vi "opt_power.vi"(11 "file path 2":path=path "C:/luminartech/ManufacturingTools/TS_Automation/Programs/Labview/bring_up/find_opt_power/opt_power_resp.txt") -> (3 "opt_power":dbl)   [LabVIEW 2018]
panel:
  out "size(s)":i32
  out "text 2":string[](array[string])
  out "line 2":string
  out "data table":dbl[][](array[numeric])
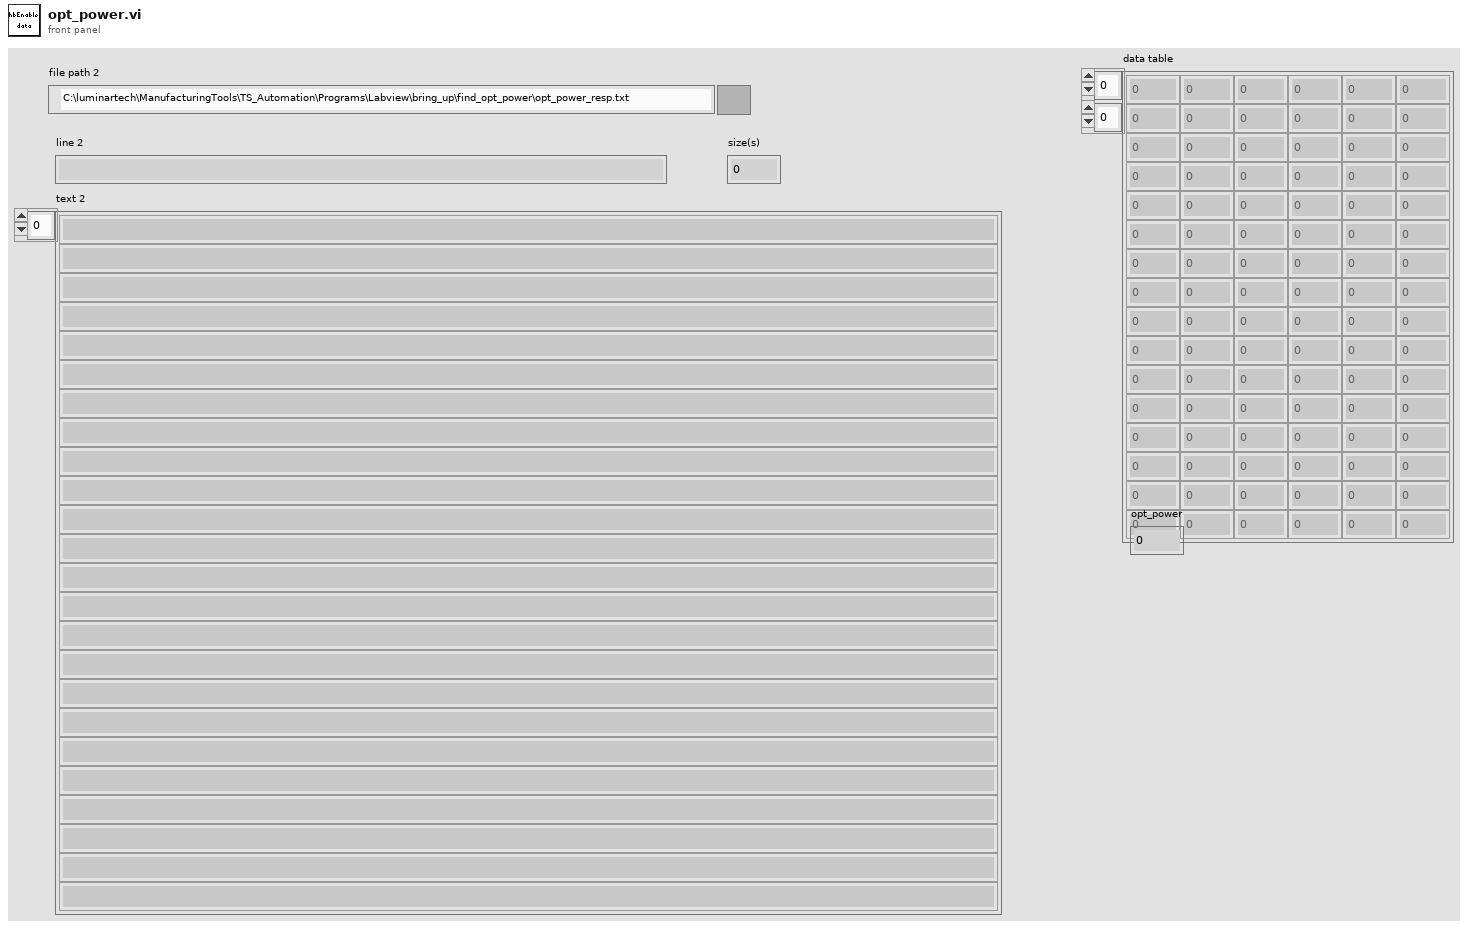
[diagram p1: front panel]
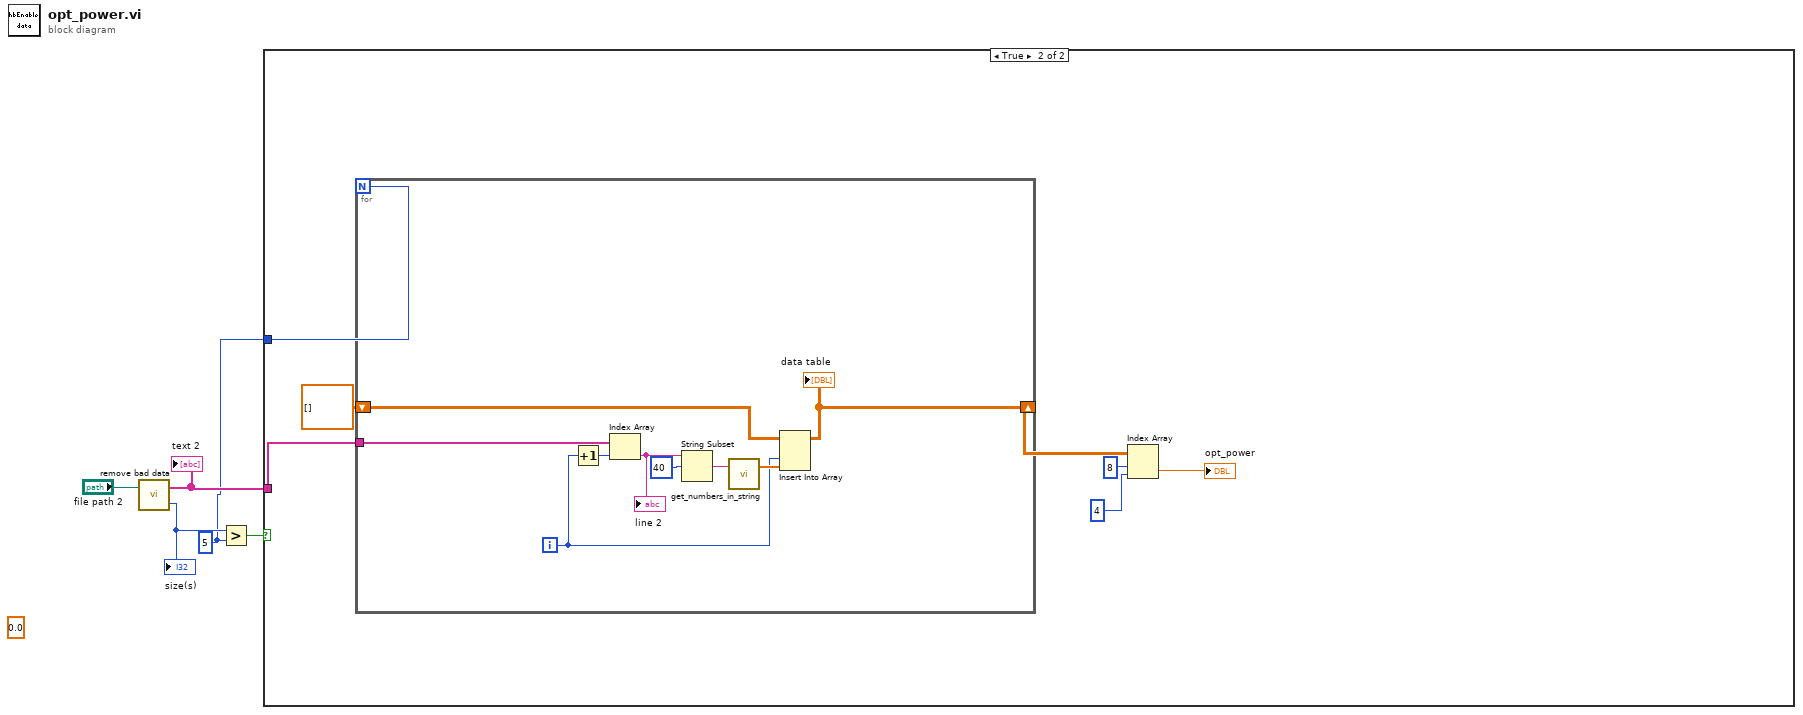
[diagram p0: block diagram]
diagram:
  (unwired) 0.0 ("COOL")
  w1 = 5 ("y")
  n1 = call "remove bad data.vi"("file path"="file path 2") -> ("size(s)"=w2:i32, "text 2"=w3:string[])  [unwired: 1 in]
  "text 2" <- w3
  "size(s)" <- w2
  n2 = Greater?(x=w2, y=w1) -> (0:w4:bool)
  n3 = case shown="True" w4 {
    tunnel: w3 -> [_ w11]
    tunnel: w1 -> [_ w10]
    frame False {
    }
    frame True {
      n4 = for {
        N: w10 -> [_]
        shift-right: [w17] -> w8
        shift-left: dbl[][] [] -> [w18]
        tunnel: w11 -> [w14]
        i -> [w15]
        n5 = Increment(x=w15) -> (x+1=w21:i32)
        n6 = Index Array(array=w14, index=w21) -> (element=w13:string)
        "line 2" <- w13
        n7 = String Subset(string=w13, offset (0)=40) -> (substring=w19:string)  [unwired: 1 in]
        n8 = call "get_numbers_in_string.vi"("String"=w19) -> ("Extracted Numbers"=w16:dbl[])  [unwired: 1 in, 1 out]
        n9 = Insert Into Array(array=w18, index (col)=w15, new element=w16) -> (w17:dbl[][])  [unwired: 1 in]
        "data table" <- w17
      }
      n10 = Index Array(array=w8, index (row)=8, index (col)=4 ("disabled index (col)")) -> (element=→"opt_power":dbl)
    }
  }
